vi "FPGA Secondary Digitize and Protect.vi"() -> ()   [LabVIEW 2020]
doc: "Author: Scott Hannahs <sth@magnet.fsu.edu>\nCopyright 2018 Florida State University, All rights reserved."
uses:
  SCH Test Controls/SCH CoWound Geometric Factor.ctl
  SCH Scaling Controls/SCH CoWound Scale Factor.ctl
  SCH Data Controls/SCH CoWound Volt Array.ctl
  SCH Data Controls/SCH Data 2 RT.ctl
  SCH Data Controls/SCH Data 2 RT Array Secondary.ctl
  SCH Test Controls/SCH CoWound Volt Limit.ctl
  SCH Data Controls/SCH Raw Int Data Secondary.ctl
  SCH Scaling Controls/SCH Dump Resistor Scale Factor.ctl
  SCH Data Controls/Digitizer State Enum.ctl
  <vilib>/rvi/Emulation/niFpgaGetClockAttributes.vi
  <vilib>/rvi/Emulation/niFpgaSctlEmulationGetInTimedLoop.vi
  <vilib>/rvi/Emulation/niFpgaEmulationReportErrorSimple.vi
  <vilib>/rvi/Emulation/niFpgaProcessEmulError.vi
  <vilib>/rvi/Emulation/niFpgaEmulationIsFPGAContextNoSignature.vi
  <vilib>/rvi/errors/niFpgaSetErrorForExecOnDevCompSimple.vi
  <vilib>/rvi/eio/common/nirviEmuReportErrorAndStop.vi
  <vilib>/rvi/DataTransferAndStorage/Container/Common/niFpgaContainerGetUniqueNameForEmu.vi
  <vilib>/rvi/FIFO/Fifo_Resource/nirvififoEmulationSetSize.vi
  <vilib>/rvi/FIFO/Fifo_Resource/nirviFifoEmulationQueueMgr.vi
  <instcachedir>/0/nirviFifoEmulationQueueMgr_E5CAEC123FF24DC58D834DCA3CDAA9B5.lvgen/nirviFifoEmulationQueueMgr_E5CAEC123FF24DC58D834DCA3CDAA9B5_007.vi
  <vilib>/Utility/error.llb/Clear Errors.vi
  <vilib>/rvi/FIFO/Fifo_Resource/nirvififoEmulationCreateLock.vi
  <vilib>/rvi/FIFO/Fifo_Resource/nirvififoEmulationObtainLock.vi
  <vilib>/rvi/FIFO/Fifo_Resource/nirvififoEmulationReleaseLock.vi
  <vilib>/rvi/occurrence/nirviWaitOnOccurrenceBase.vi
  <vilib>/rvi/errors/nirviReportUnexpectedCaseInternalError.vi
  <vilib>/rvi/errors/nirviReportUnexpectedCaseInternalError (U32).vi
  <vilib>/rvi/Emulation/niFpgaCriticalErrorInLSC.vi
  <vilib>/rvi/eio/common/nirviEmuTemplateMethod_errors.vi
  <vilib>/rvi/FIFO/Fifo_Resource/nirvififoEmulationDetermineInputValidOut.vi
  <vilib>/rvi/DataTransferAndStorage/Container/XNode/niFpgaContainer.xnode
  <vilib>/rvi/FIFO/Fifo_Resource/nirvififoEmulationRead.vi
  <vilib>/eio/EIONode/EIONode.xnode
  <vilib>/rvi/FIFO/Fifo_Resource/nirvififoEmulationWrite.vi
  <vilib>/rvi/interface/RandomDataEmulation/nirviRandomDataFpgaReadWriteTemplate.vi
panel:
  out "Build":u8=64
  out "Fix":u8=3
  out "Minor":u8=2
  out "Major":u8=2
  out "Current":T1 format="%.4f"
  out "Overall WDT":bool
  out "DAQ Loop WDT OK":bool
  out "Co-Wound Loop WDT OK":bool
  out "PS Enable Loop WDT OK":bool
  out "Breaker Enable":bool
  out "Low Current Mode":bool
  out "DAQ Zero Fault":bool
  out "Co-Wound Index":i32
  out "Read Error Index":i32
  out "Calibrate Loop Index":i32
  out "PS Enable Index":i32
  out "Watch Dog Index":i32
  out "Digitizer Read OK":bool
  in  "Input Select":T2(ring)
  in  "Tab Control":T3(tab)
  out "CoWound Volt Array":T4 format="%.4f"
  in  "Co-Wound Scale Factor":T5=59.95204000174999
  in  "Co-Wound Asymmetry Factor":T6=-0.0026702880859375 format="%.8g"
  in  "Cold Mass Scale Factor":T7=59.98800000548363
  out "Co-Wound Error":fxp<+,38,12> format="%.4f"
  out "Offset":T8
  out "Calibrate Index":i16
  out "Scale":T8
  in  "Current Scale Factor":T1=2.0 format="%_6g"
  in  "Low Current Delay Factor":u16=100
  in  "Low Current Ticks":u32=400000000
  in  "Low Current (kA)":T1=0.04500000178813934 format="%_6g"
  in  "Digitize # Bits":u32=16
  in  "Digitize Read Delay Ticks":u32=41
  in  "Convert Clock Ticks":u32=20
  in  "Digitize Reset Ticks":u32=400
  in  "DAQ Cycle Ticks":u32=4096
  in  "CoWound Tick Limit":u32=4000000
  in  "CoWound Volt Limit":T9=0.20001220703125
  out "Data Size":i32
  in  "Ln2 Filter Size":i16=10
  out "Chassis Temperature":fxp<+/-,16,14> format="%.2f"
  in  "# Consecutive Zeros Fault":i16=1000
  in  "Digitize Convert Ticks":u32=200
  out "uSec/Cycle":u32
  out "Proto Co-Wournd Limit":bool
  out "Co-Wound Limit Err":bool
  out "Breaker First Error":u64 format="%010x"
  out "Timed Out? FIFO Raw":bool
  out "Timed Out? FIFO2RT Filter":bool
  out "Timed Out? Co-Wound Read":bool
  out "Timed Out? FIFO2RT Raw":bool
  out "DAQ Zero Fault Channel":bool[](array[boolean])
  out "DAQ Loop WDT":bool
  out "Co-Wound Loop WDT":bool
  out "PS Enable Loop WDT":bool
  out "Raw Data":T10 format="%.4p"
  out "Filt Data":T10 format="%.4p"
  in  "Stop WD Loop":bool
  out "16 Bit Digitizer output":T8
  in  "Reset":bool
  in  "stop":bool
  out "Main Index":i32
  # "."
  # "."
  # "."
  # "Cold Mass Voltage"
  # "Co-Wound Voltage"
  # "`"
  # "SCH Protection Globals"
  # "All Clock Ticks are at 40 MHz"
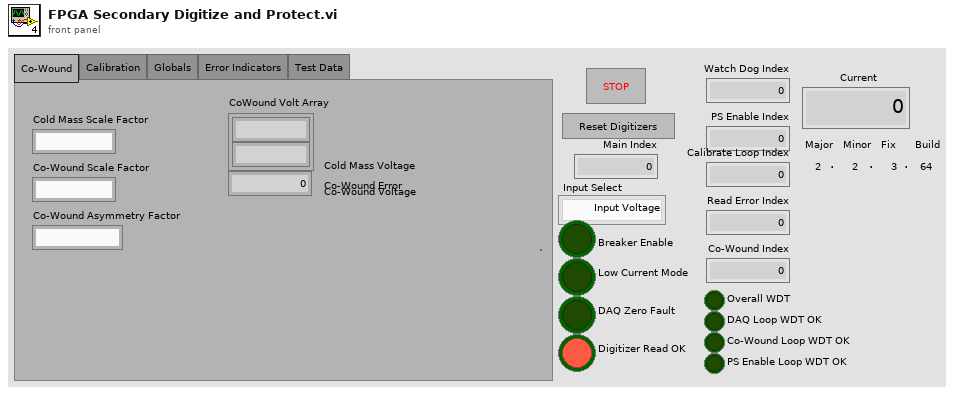
[diagram p1: front panel]
types:
  T1 = typedef "SCH Data 2 RT.ctl" = fxp<+/-,38,12>
  T2 = enum16{"Input Voltage", "Zero Voltage", "Calibrate Voltage"}
  T3 = enum32{"Co-Wound", "Calibration", "Globals", "Error Indicators", "Test Data"}
  T4 = typedef "SCH CoWound Volt Array.ctl" = T1[]
  T5 = typedef "SCH CoWound Scale Factor.ctl" = fxp<+/-,38,12>
  T6 = typedef "SCH CoWound Geometric Factor.ctl" = fxp<+/-,16,0>
  T7 = typedef "SCH Dump Resistor Scale Factor.ctl" = fxp<+/-,38,12>
  T8 = typedef "SCH Raw Int Data Secondary.ctl" = i16[]
  T9 = typedef "SCH CoWound Volt Limit.ctl" = fxp<+/-,16,1>
  T10 = typedef "SCH Data 2 RT Array Secondary.ctl" = T1[]
  T11 = typedef "Digitizer State Enum.ctl" = enum16{"Reset", "StartCnvt"}
  T12 = typedef "SCH Secondary Int Data.ctl" = fxp<+/-,19,5>[]
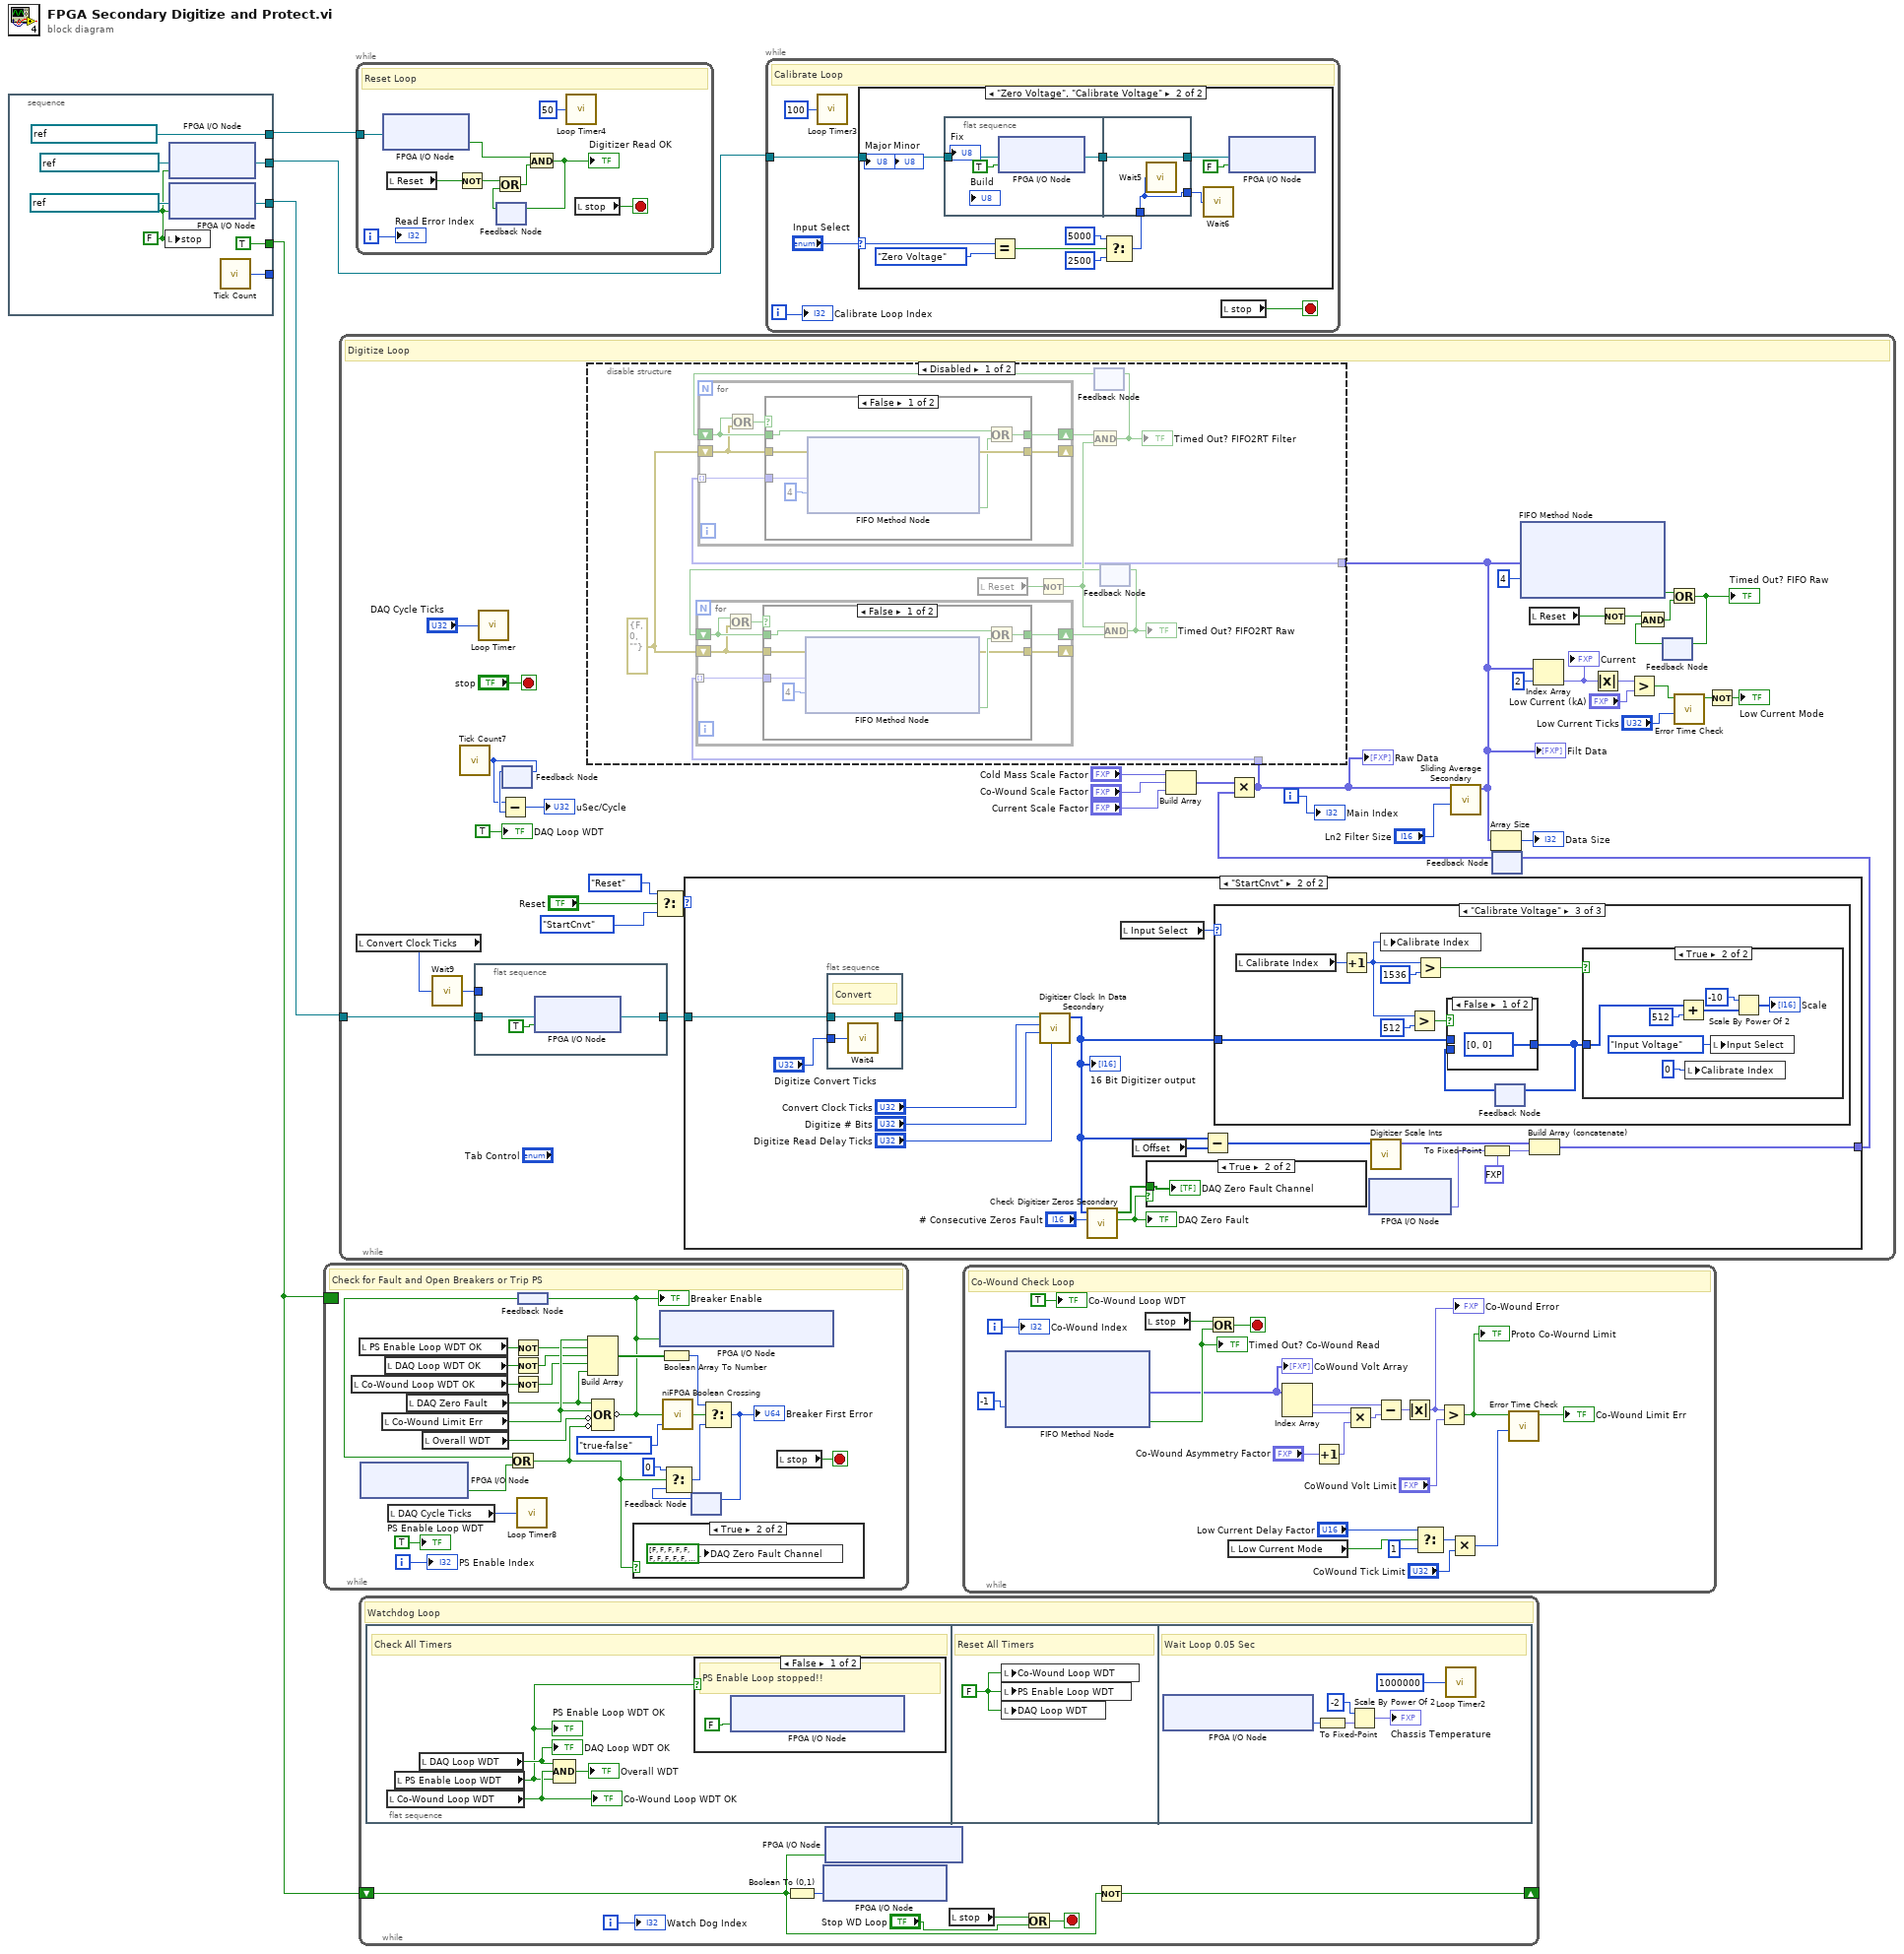
[diagram p0: block diagram]
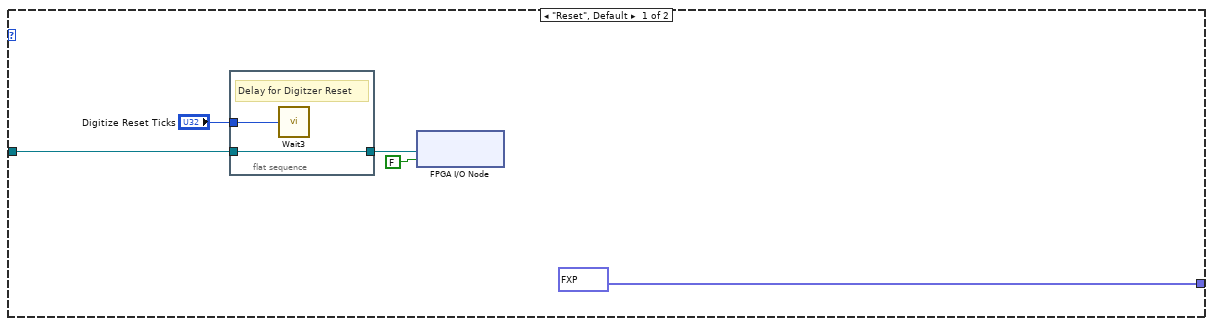
[diagram p7: hidden frame]
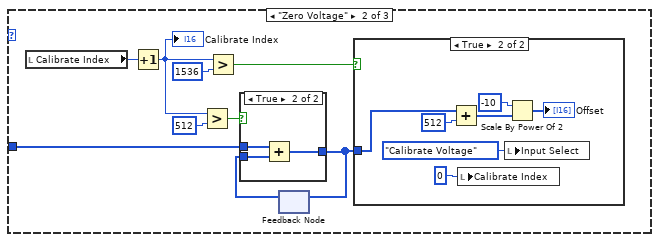
[diagram p10: hidden frame]
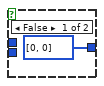
[diagram p12: hidden frame]
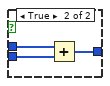
[diagram p14: hidden frame]
diagram:
  n1 = stacked-sequence {
    tunnel: [w12] -> w4
    tunnel: [TRUE] -> w3
    tunnel: [w9] -> _
    tunnel: [w6] -> w2
    tunnel: [refnum<k21> "Digitizer Read Error" ("FPGA I/O In")] -> w1
    frame #0 {
      w7 = FALSE ("Connector0/DIO0")
      n2 = local write "stop"(w7) -> ()
      n3 = xnode "FPGA I/O Node"("I/O Item"=w7, "FPGA I/O In"=refnum<k21> "Digitizer Calibrate") -> ("FPGA I/O Out"=w6:refnum<k21>)
      n4 = xnode "FPGA I/O Node"("I/O Item"=w7, "FPGA I/O In"=refnum<k21> "Digitizer Clock Data") -> ("FPGA I/O Out"=w12:refnum<k21>)
      n5 = call "Tick Count"() -> ("Tick Count(Ticks)"=w9:u32)
    }
  }
  n6 = while {
    border: w3 -> [_]
    i -> [w19]
    stop <- w37 stop-if-true
    # "Check for Fault and Open Breakers or Trip PS"
    n7 = local read "Co-Wound Loop WDT OK"() -> (w29:bool)
    n8 = local read "PS Enable Loop WDT OK"() -> (w30:bool)
    n9 = xnode "FPGA I/O Node"() -> ("Reset Switch"=w17:bool)  [unwired: 1 in, 1 out]
    n10 = local read "Co-Wound Limit Err"() -> (w34:bool)
    n11 = local read "DAQ Loop WDT OK"() -> (w22:bool)
    n12 = local read "DAQ Cycle Ticks"() -> (w18:u32)
    n13 = local read "DAQ Zero Fault"() -> (w15:bool)
    n14 = local read "Overall WDT"() -> (w14:bool)
    n15 = Not(x=w30) -> (.not. x?=w23:bool)
    n16 = Not(x=w22) -> (.not. x?=w21:bool)
    n17 = Not(x=w29) -> (.not. x?=w20:bool)
    n18 = call "Loop Timer8"("Count(Ticks)"=w18) -> ()  [unwired: 1 out]
    n19 = feedback #1() -> (w33:bool)
    n20 = Or(x=w33, y=w17) -> (x .or. y?=w13:bool)
    n21 = Build Array(w34, w23, w21, w20, w15) -> (w31:bool[])
    n22 = Compound Arithmetic op=OR(w15, w34, invert w14, invert w13) -> (invert w16:bool)
    "Breaker Enable" <- w16
    n23 = feedback-in #1(w16) -> ()
    n24 = case shown="True" w13 {
      frame False {
      }
      frame True {
        n25 = local write "DAQ Zero Fault Channel"(bool[] [FALSE, FALSE, FALSE, FALSE, FALSE, FALSE, FALSE, FALSE, FALSE, FALSE, FALSE, FALSE, FALSE, FALSE, FALSE, FALSE, FALSE, FALSE, FALSE, FALSE, FALSE, FALSE, FALSE, FALSE, FALSE, FALSE, FALSE, FALSE, FALSE, FALSE, FALSE, FALSE, FALSE, FALSE, FALSE, FALSE, FALSE, FALSE] ("DAQ Fault Channel")) -> ()
      }
    }
    n26 = xnode "FPGA I/O Node"("SCHMPS2 Breaker Enable"=w16) -> ()  [unwired: 1 in, 1 out]
    n27 = Boolean Array To Number(Boolean array=w31) -> (number=w27:u8)
    n28 = call <vilib>:"niFPGA Boolean Crossing.vi"("input"=w16, "direction"=enum8{"either", "false-true", "true-false"}."true-false") -> ("crossing"=w28:bool)  [unwired: 7 in]
    n29 = feedback #2() -> (w25:u64)  [unwired: 1 in]
    n30 = Select(t=u64 0, s=w13, f=w25) -> (s? t:f=w24:u64)
    n31 = Select(t=w27, s=w28, f=w24) -> (s? t:f=w26:u64)
    "Breaker First Error" <- w26
    n32 = feedback-in #2(w26) -> ()
    n33 = local read "stop"() -> (w37:bool)
    "PS Enable Loop WDT" <- TRUE
    "PS Enable Index" <- w19
  }
  n34 = while {
    tunnel: w4 -> [w74]
    i -> [w65]
    stop <- "stop" stop-if-true
    # "Digitize Loop"
    n35 = local read "Convert Clock Ticks"() -> (w52:u32)
    n36 = call "Wait9"("Count(Ticks)"=w52) -> ("Tick Count(Ticks)"=w75:u32)
    n37 = call "Tick Count7"() -> ("Tick Count(uSec)"=w68:u32)
    n38 = flat-sequence {
      tunnel: w75 -> [_]
      tunnel: w74 -> [w121]
      tunnel: [w120] -> w73
      frame #0 {
        n39 = xnode "FPGA I/O Node"("I/O Item"=TRUE ("Connector0/DIO0"), "FPGA I/O In"=w121) -> ("FPGA I/O Out"=w120:refnum<k21>)
      }
    }
    n40 = call "Loop Timer"("Count(Ticks)"="DAQ Cycle Ticks") -> ()  [unwired: 1 out]
    n41 = feedback #3() -> (w69:u32)  [unwired: 1 in]
    n42 = Subtract(x=w68, y=w69) -> (x-y=→"uSec/Cycle":u32)
    n43 = feedback-in #3(w68) -> ()
    n44 = Select(t=Digitizer_State_Enum."Reset", s="Reset", f=Digitizer_State_Enum."StartCnvt" ("t")) -> (s? t:f=w76:T11)
    n45 = case shown="\"StartCnvt\"" w76 {
      tunnel: w73 -> [w125 w147]
      tunnel: [fxp<+/-,19,5>[] [0.0, 0.0, 0.0] ("Array") w133] -> w70
      frame "Reset", Default {
        n46 = flat-sequence {
          tunnel: [w129] -> w126
          tunnel: w125 -> [w129]
          tunnel: "Digitize Reset Ticks" -> [w128]
          frame #0 {
            # "Delay for Digitzer Reset"
            n47 = call "Wait3"("Count(Ticks)"=w128) -> ()  [unwired: 1 out]
          }
        }
        n48 = xnode "FPGA I/O Node"("I/O Item"=FALSE ("Connector0/DIO0"), "FPGA I/O In"=w126) -> ()  [unwired: 1 out]
      }
      frame "StartCnvt" {
        n49 = flat-sequence {
          tunnel: [w190] -> w146
          tunnel: w147 -> [w190]
          tunnel: "Digitize Convert Ticks" -> [w189]
          frame #0 {
            # "Convert"
            n50 = call "Wait4"("Count(Ticks)"=w189) -> ()  [unwired: 1 out]
          }
        }
        n51 = call "Digitizer Clock In Data Secondary.vi"("Digitize Read Delay Ticks"="Digitize Read Delay Ticks", "Digitize # Bits"="Digitize # Bits", "Convert Clock Ticks"="Convert Clock Ticks", "Refnum in"=w146) -> ("Data Out"=w139:T8)  [unwired: 7 in]
        "16 Bit Digitizer output" <- w139
        n52 = call "Check Digitizer Zeros Secondary.vi"("# Consecutive Zeros Fault"="# Consecutive Zeros Fault", "DAQ Raw Data"=w139) -> ("DAQ Zero Fault"=w141:bool, "DAQ Zero Fault Channel"=w143:bool[])  [unwired: 8 in]
        "DAQ Zero Fault" <- w141
        n53 = local read "Input Select"() -> (w144:T2)
        n54 = local read "Offset"() -> (w145:T8)
        n55 = case shown="True" w141 {
          tunnel: w143 -> [_ w148]
          frame False {
          }
          frame True {
            "DAQ Zero Fault Channel" <- w148
          }
        }
        n56 = Subtract(x=w139, y=w145) -> (x-y=w135:T8)
        n57 = case shown="\"Calibrate Voltage\"" w144 {
          tunnel: w139 -> [_ w154 w174]
          frame "Input Voltage", Default {
          }
          frame "Zero Voltage" {
            n58 = local read "Calibrate Index"() -> (w156:i16)
            n59 = Increment(x=w156) -> (x+1=w149:i16)
            "Calibrate Index" <- w149
            n60 = Greater?(x=w149, y=i16 512) -> (0:w155:bool)
            n61 = Greater?(x=w149, y=i16 1536) -> (0:w152:bool)
            n62 = feedback #4() -> (w150:i32[])  [unwired: 1 in]
            n63 = case shown="True" w155 {
              tunnel: w154 -> [_ w168]
              tunnel: [T8 [0, 0] ("16 Bit Digitizer output") w167] -> w151
              tunnel: w150 -> [_ w166]
              frame False {
              }
              frame True {
                n64 = Add(x=w168, y=w166) -> (x+y=w167:i32[])
              }
            }
            n65 = feedback-in #4(w151) -> ()
            n66 = case shown="True" w152 {
              tunnel: w151 -> [_ w163]
              frame False {
              }
              frame True {
                n67 = Add(x=w163, y=512 ("n")) -> (x+y=w159:i32[])
                n68 = local write "Calibrate Index"(i16 0 ("Calibrate Index")) -> ()
                n69 = local write "Input Select"(T2."Calibrate Voltage" ("Input Select")) -> ()
                n70 = Scale By Power Of 2(n=i16 -10, x=w159) -> (x*2^n=→"Offset":i32[])
              }
            }
          }
          frame "Calibrate Voltage" {
            n71 = local read "Calibrate Index"() -> (w176:i16)
            n72 = Increment(x=w176) -> (x+1=w169:i16)
            n73 = local write "Calibrate Index"(w169) -> ()
            n74 = Greater?(x=w169, y=i16 512) -> (0:w175:bool)
            n75 = Greater?(x=w169, y=i16 1536) -> (0:w172:bool)
            n76 = feedback #5() -> (w170:i32[])  [unwired: 1 in]
            n77 = case shown="False" w175 {
              tunnel: w174 -> [_ w188]
              tunnel: [T8 [0, 0] ("16 Bit Digitizer output") w187] -> w171
              tunnel: w170 -> [_ w186]
              frame False {
              }
              frame True {
                n78 = Add(x=w188, y=w186) -> (x+y=w187:i32[])
              }
            }
            n79 = feedback-in #5(w171) -> ()
            n80 = case shown="True" w172 {
              tunnel: w171 -> [_ w183]
              frame False {
              }
              frame True {
                n81 = Add(x=w183, y=512 ("n")) -> (x+y=w179:i32[])
                n82 = local write "Calibrate Index"(i16 0 ("Calibrate Index")) -> ()
                n83 = local write "Input Select"(T2."Input Voltage" ("Input Select")) -> ()
                n84 = Scale By Power Of 2(n=i16 -10, x=w179) -> (x*2^n=→"Scale":i32[])
              }
            }
          }
        }
        n85 = xnode "FPGA I/O Node"() -> ("Current"=w131:fxp<+/-,24,5>)  [unwired: 1 in, 1 out]
        n86 = call "Digitizer Scale Ints.vi"("Data Out"=w135) -> ("Array"=w134:T12)  [unwired: 10 in]
        n87 = To Fixed-Point(fixed-point type=fxp<+/-,19,5> 0.0, number=w131) -> (fixed-point=w132:fxp<+/-,19,5>)
        n88 = Build Array (concatenate)(w134, w132) -> (w133:fxp<+/-,19,5>[])
      }
    }
    n89 = Build Array("Cold Mass Scale Factor", "Co-Wound Scale Factor", "Current Scale Factor") -> (w66:T1[])
    n90 = feedback-in #6(w70) -> ()
    n91 = feedback #6() -> (w61:fxp<+/-,19,5>[])  [unwired: 1 in]
    n92 = Multiply(x=w66, y=w61) -> (x*y=w50:T1[])
    "Raw Data" <- w50
    n93 = call "Sliding Average Secondary.vi"("Ln2 Filter Size"="Ln2 Filter Size", "Array In"=w50) -> ("Filtered Array Out"=w39:T10)  [unwired: 9 in]
    "Filt Data" <- w39
    n94 = disable-structure shown="Disabled" {
      disable-tunnel: w39 -> [w80 _]
      disable-tunnel: w50 -> [w79 _]
      frame Disabled {
        w82 = errorcluster {"Status?"=FALSE, "Code"=0, "Source"=""} ("error out")
        n95 = local read "Reset"() -> (w85:bool)
        n96 = Not(x=w85) -> (.not. x?=w81:bool)
        n97 = feedback #7() -> (w84:bool)  [unwired: 1 in]
        n98 = for {
          tunnel: w80 -> [w110] mode=indexing
          shift-right: [w109] -> w89
          shift-left: w84 -> [w106]
          shift-right: [w108] -> _
          shift-left: w82 -> [w105]
          n99 = Or(x=w106, y=w105) -> (x .or. y?=w107:bool)
          n100 = case shown="False" w107 {
            tunnel: w110 -> [w114 _]
            tunnel: [w117 w118] -> w109
            tunnel: w106 -> [w116 w118]
            tunnel: w105 -> [w113 w119]
            tunnel: [w112 w119] -> w108
            frame False {
              n101 = xnode ("FIFO Method Node")("Element"=w114, "Timeout"=4, "error in (no error)"=w113) -> ("Timed Out?"=w111:bool, "error out"=w112:errorcluster)  [unwired: 1 in, 1 out]
              n102 = Or(x=w116, y=w111) -> (x .or. y?=w117:bool)
            }
            frame True {
            }
          }
        }
        n103 = And(x=w89, y=w81) -> (x .and. y?=w88:bool)
        "Timed Out? FIFO2RT Filter" <- w88
        n104 = feedback-in #7(w88) -> ()
        n105 = feedback #8() -> (w83:bool)  [unwired: 1 in]
        n106 = for {
          tunnel: w79 -> [w95] mode=indexing
          shift-right: [w94] -> w86
          shift-left: w83 -> [w92]
          shift-right: [w93] -> _
          shift-left: w82 -> [w91]
          n107 = Or(x=w92, y=w91) -> (x .or. y?=w90:bool)
          n108 = case shown="False" w90 {
            tunnel: w95 -> [w102 _]
            tunnel: [w100 w103] -> w94
            tunnel: w92 -> [w99 w103]
            tunnel: w91 -> [w97 w104]
            tunnel: [w96 w104] -> w93
            frame False {
              n109 = xnode ("FIFO Method Node")("Element"=w102, "Timeout"=4, "error in (no error)"=w97) -> ("Timed Out?"=w101:bool, "error out"=w96:errorcluster)  [unwired: 1 in, 1 out]
              n110 = Or(x=w99, y=w101) -> (x .or. y?=w100:bool)
            }
            frame True {
            }
          }
        }
        n111 = And(x=w81, y=w86) -> (x .and. y?=w87:bool)
        "Timed Out? FIFO2RT Raw" <- w87
        n112 = feedback-in #8(w87) -> ()
      }
      frame Enabled {
      }
    }
    n113 = Array Size(array=w39) -> (size(s)=→"Data Size":i32)
    n114 = xnode ("FIFO Method Node")("Element"=w39, "Timeout"=4) -> ("Timed Out?"=w59:bool)  [unwired: 1 in, 1 out]
    n115 = local read "Reset"() -> (w56:bool)
    n116 = Index Array(array=w39, index=2) -> (element=w43:T1)
    "Current" <- w43
    n117 = Absolute Value(x=w43) -> (abs(x)=w42:fxp<+,38,12>)
    n118 = Not(x=w56) -> (.not. x?=w55:bool)
    n119 = Greater?(x=w42, y="Low Current (kA)") -> (0:w45:bool)
    n120 = feedback #9() -> (w58:bool)  [unwired: 1 in]
    n121 = And(x=w55, y=w58) -> (x .and. y?=w57:bool)
    n122 = Or(x=w59, y=w57) -> (x .or. y?=w54:bool)
    "Timed Out? FIFO Raw" <- w54
    n123 = feedback-in #9(w54) -> ()
    n124 = call "Error Time Check.vi"("Ticks Until Trigger"="Low Current Ticks", "Limit Exceeded"=w45) -> ("Limit Triggered"=w44:bool)  [unwired: 9 in]
    n125 = Not(x=w44) -> (.not. x?=→"Low Current Mode":bool)
    "Main Index" <- w65
    "DAQ Loop WDT" <- TRUE ("DAQ Loop WDT")
  }
  n126 = while {
    tunnel: w1 -> [w199]
    i -> [w192]
    stop <- w200 stop-if-true
    # "Reset Loop"
    n127 = xnode "FPGA I/O Node"("FPGA I/O In"=w199) -> ("I/O Item"=w198:bool)  [unwired: 1 out]
    n128 = local read "Reset"() -> (w194:bool)
    n129 = Not(x=w194) -> (.not. x?=w193:bool)
    n130 = feedback #10() -> (w196:bool)  [unwired: 1 in]
    n131 = Or(x=w193, y=w196) -> (x .or. y?=w195:bool)
    n132 = And(x=w198, y=w195) -> (x .and. y?=w197:bool)
    "Digitizer Read OK" <- w197
    n133 = feedback-in #10(w197) -> ()
    n134 = call "Loop Timer4"("Count(uSec)"=u32 50) -> ()  [unwired: 1 out]
    n135 = local read "stop"() -> (w200:bool)
    "Read Error Index" <- w192
  }
  n136 = while {
    shift-right: [w206] -> _
    shift-left: w3 -> [w201]
    i -> [w202]
    stop <- w204 stop-if-true
    # "Watchdog Loop"
    n137 = flat-sequence {
      frame #0 {
        # "Check All Timers"
        n138 = local read "Co-Wound Loop WDT"() -> (w209:bool)
        "Co-Wound Loop WDT OK" <- w209
        n139 = local read "PS Enable Loop WDT"() -> (w208:bool)
        "PS Enable Loop WDT OK" <- w208
        n140 = local read "DAQ Loop WDT"() -> (w210:bool)
        "DAQ Loop WDT OK" <- w210
        n141 = Compound Arithmetic op=AND(w210, w209, w208) -> (→"Overall WDT":bool)
        n142 = case shown="False" w208 {
          frame False {
            # "PS Enable Loop stopped!!"
            n143 = xnode "FPGA I/O Node"("SCHMPS2 Breaker Enable"=FALSE ("Calc Loop WDT")) -> ()  [unwired: 1 in, 1 out]
          }
          frame True {
          }
        }
      }
      frame #1 {
        w213 = FALSE ("Calc Loop WDT")
        # "Reset All Timers"
        n144 = local write "Co-Wound Loop WDT"(w213) -> ()
        n145 = local write "PS Enable Loop WDT"(w213) -> ()
        n146 = local write "DAQ Loop WDT"(w213) -> ()
      }
      frame #2 {
        # "Wait Loop 0.05 Sec"
        n147 = xnode "FPGA I/O Node"() -> ("Chassis Temperature"=w217:i16)  [unwired: 1 in, 1 out]
        n148 = To Fixed-Point(number=w217) -> (fixed-point=w214:fxp<+/-,16,14>)  [unwired: 1 in]
        n149 = Scale By Power Of 2(n=i16 -2 ("Chassis Temperature"), x=w214) -> (x*2^n=→"Chassis Temperature":fxp<+/-,16,14>)
        n150 = call "Loop Timer2"("Count(Ticks)"=u32 1000000) -> ()  [unwired: 1 out]
      }
    }
    n151 = Boolean To (0,1)(Boolean=w201) -> (0, 1=w205:i16)
    n152 = xnode "FPGA I/O Node"("USER FPGA LED"=w205) -> ()  [unwired: 1 in, 1 out]
    n153 = xnode "FPGA I/O Node"("Watchdog Output"=w201) -> ()  [unwired: 1 in, 1 out]
    n154 = local read "stop"() -> (w207:bool)
    n155 = Or(x=w207, y="Stop WD Loop") -> (x .or. y?=w204:bool)
    n156 = Not(x=w201) -> (.not. x?=w206:bool)
    "Watch Dog Index" <- w202
  }
  n157 = while {
    tunnel: w2 -> [w222]
    i -> [w220]
    stop <- w221 stop-if-true
    # "Calibrate Loop"
    n158 = call "Loop Timer3"("Count(uSec)"=u32 100) -> ()  [unwired: 1 out]
    n159 = case shown="\"Zero Voltage\", \"Calibrate Voltage\"" "Input Select" {
      selector: "Input Select" -> [_ w234]
      tunnel: w222 -> [_ w229]
      frame "Input Voltage", Default {
      }
      frame "Zero Voltage", "Calibrate Voltage" {
        n160 = flat-sequence {
          tunnel: w229 -> [w236]
          tunnel: [w235] -> w227
          tunnel: w228 -> [w238]
          tunnel: w227 -> [w239]
          tunnel: [w239] -> w226
          tunnel: [w238] -> w224
          frame #0 {
            n161 = xnode "FPGA I/O Node"("I/O Item"=TRUE ("Connector0/DIO0"), "FPGA I/O In"=w236) -> ("FPGA I/O Out"=w235:refnum<k21>)
          }
          frame #1 {
            n162 = call "Wait5"("Count(uSec)"=w238) -> ()  [unwired: 1 out]
          }
        }
        n163 = Equal?(x=w234, y=T2."Zero Voltage") -> (x = y?=w232:bool)
        n164 = Select(t=u16 5000 ("Count(uSec)"), s=w232, f=u16 2500 ("Count(uSec)")) -> (s? t:f=w228:u16)
        n165 = call "Wait6"("Count(uSec)"=w224) -> ()  [unwired: 1 out]
        n166 = xnode "FPGA I/O Node"("I/O Item"=FALSE ("Connector0/DIO0"), "FPGA I/O In"=w226) -> ()  [unwired: 1 out]
      }
    }
    n167 = local read "stop"() -> (w221:bool)
    "Calibrate Loop Index" <- w220
  }
  n168 = while {
    i -> [w250]
    stop <- w255 stop-if-true
    # "Co-Wound Check Loop"
    n169 = xnode ("FIFO Method Node")("Timeout"=-1) -> ("Element"=w252:fxp<+/-,38,12>[], "Timed Out?"=w254:bool)  [unwired: 1 in, 1 out]
    "Timed Out? Co-Wound Read" <- w254
    "CoWound Volt Array" <- w252
    n170 = local read "stop"() -> (w256:bool)
    n171 = Or(x=w256, y=w254) -> (x .or. y?=w255:bool)
    n172 = local read "Low Current Mode"() -> (w243:bool)
    n173 = Index Array(array=w252) -> (element #1=w259:fxp<+/-,38,12>, element #2=w261:fxp<+/-,38,12>)  [unwired: 2 in]
    n174 = Increment(x="Co-Wound Asymmetry Factor") -> (x+1=w251:fxp<+,17,1>)
    n175 = Multiply(x=w261, y=w251) -> (x*y=w260:fxp<+/-,54,12>)
    n176 = Subtract(x=w259, y=w260) -> (x-y=w258:fxp<+/-,38,12>)
    n177 = Absolute Value(x=w258) -> (abs(x)=w240:fxp<+,38,12>)
    "Co-Wound Error" <- w240
    n178 = Select(t="Low Current Delay Factor", s=w243, f=u16 1) -> (s? t:f=w249:u16)
    n179 = Greater?(x=w240, y="CoWound Volt Limit") -> (0:w244:bool)
    "Proto Co-Wournd Limit" <- w244
    n180 = Multiply(x=w249, y="CoWound Tick Limit") -> (x*y=w247:u32)
    n181 = call "Error Time Check.vi"("Ticks Until Trigger"=w247, "Limit Exceeded"=w244) -> ("Limit Triggered"=→"Co-Wound Limit Err":bool)  [unwired: 9 in]
    "Co-Wound Loop WDT" <- TRUE ("Co-Wound Loop WDT")
    "Co-Wound Index" <- w250
  }
